vi "Set Initialization Data - UI Cam 2.vi"(8 "error in":errorcluster, 10 "Container":refnum<class "MDI Container.lvclass">, 11 "Container in":refnum<class "Container.lvclass">) -> (0 "error out":errorcluster, 3 "Container out":refnum<class "Container.lvclass">)   [LabVIEW 2023, in "Container.lvclass"]
doc: "Sets the initialization data of a statically linked subWorker."
uses:
  Container.lvclass
  <vilib>/MGI/Panel Manager - .NET Panels/MDI/MDI Container/MDI Container.lvclass
  UI Cam Basler/Initialization Data.ctl
  <vilib>/MGI/Panel Manager/Panel/Window Position/Reference Position/Alignment.ctl
  <vilib>/MGI/Panel Manager/Panel/Window Position/Reference Position/Horizontal Alignment.ctl
  <vilib>/MGI/Panel Manager/Panel/Window Position/Reference Position/Vertical Alignment.ctl
  Container.lvclass/Container.ctl
  UI Cam Basler/UI Cam Basler.lvclass
  C:/Program Files (x86)/National Instruments/LabVIEW 2023/vi.lib/addons/_Workers/Library/Classes/Worker/Worker.lvclass
  <vilib>/MGI/Panel Manager/Panel/Window Position/Reference Position/Reference Position.lvclass
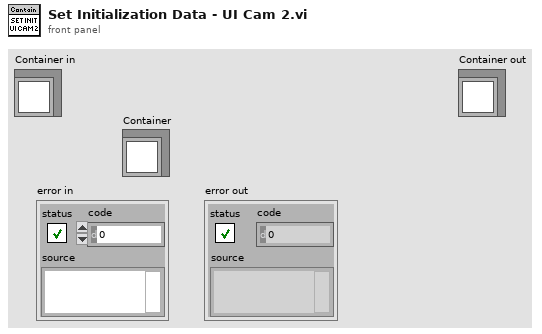
[diagram p1: front panel]
types:
  T1 = typedef "Panel.lvlib/Reference Position.lvclass/Alignment.ctl" = cluster{"Horizontal":T2, "Vertical":T3}
  T2 = typedef "Panel.lvlib/Reference Position.lvclass/Horizontal Alignment.ctl" = enum16{"Left", "Center", "Right"}
  T3 = typedef "Panel.lvlib/Reference Position.lvclass/Vertical Alignment.ctl" = enum16{"Top", "Center", "Bottom"}
  T4 = typedef "UI Cam Basler.lvclass/Initialization Data.ctl" = cluster{"Module Name":string, "Container":refnum<class "MDI Container.lvclass">, "Offset":cluster{"Horizontal":i16, "Vertical":i16}, "Width Scale":dbl, "Height Scale":dbl, "Alignment":T1}
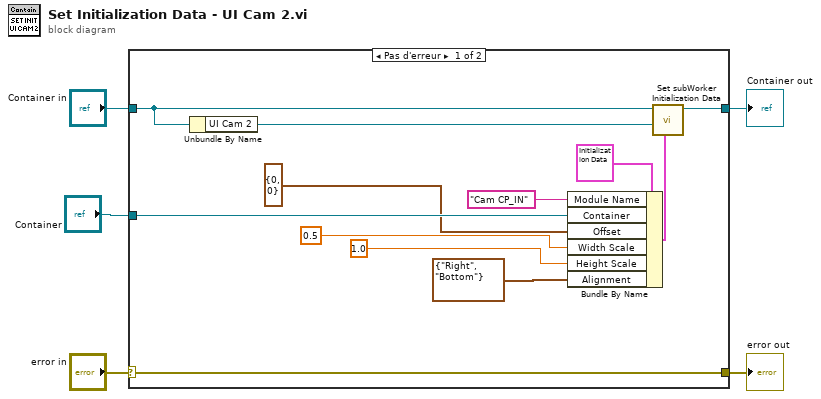
[diagram p0: block diagram]
diagram:
  n1 = case shown="Pas d'erreur" "error in" {
    selector: "error in" -> [w17 w19]
    tunnel: [w17 w19] -> w4
    tunnel: [w15 w18] -> w3
    tunnel: "Container in" -> [w14 w18]
    tunnel: "Container" -> [w10 _]
    frame No Error {
      n2 = Unbundle By Name(w14) -> ("UI Cam 2"=w16:refnum<class "UI Cam Basler.lvclass">)
      n3 = Bundle By Name(cluster=T4 {"Module Name"="", "Container"=refnum, "Offset"={"Horizontal"=0, "Vertical"=0}, "Width Scale"=300.0, "Height Scale"=500.0, "Alignment"={"Horizontal"=enum."Left", "Vertical"=enum."Top"}} ("Initialization Data"), "Module Name"="Cam CP_IN" ("Placeholder"), "Container"=w10, "Offset"=cluster{"Horizontal":i16, "Vertical":i16} {"Horizontal"=0, "Vertical"=0}, "Width Scale"=0.5, "Height Scale"=1.0, "Alignment"=T1 {"Horizontal"=enum."Right", "Vertical"=enum."Bottom"}) -> (w12:T4)
      n4 = call-dynamic "Set subWorker Initialization Data.vi"("Initialization Data"=w12, "subWorker"=w16, "Worker"=w14) -> ("Worker out"=w15:refnum<class "Container.lvclass">)  [unwired: 8 in]
    }
    frame Error {
    }
  }
  "error out" <- w4
  "Container out" <- w3
